vi "FaulhaberV3-Ascii_V1.vi"() -> (1 "searchnames":string[](array[string]), 2 "ID":u32[](array[numeric]), 3 "Faulhaber Objects":T3(array[cluster]))   [LabVIEW 2011] (continued)
"Default"="", "Kommentart"=""}, {"ID"=588578825, "Name"="Motor encoder_Speed filter", "type"=enum."U16", "rw"=enum."rw", "lowLimit"="0", "highLimit"="65535", "Default"="10", "Kommentart"=""}, {"ID"=588578826, "Name"="Motor encoder_Single turn position 16 bit", "type"=enum."U16", "rw"=enum."ro", "lowLimit"="", "highLimit"="", "Default"="", "Kommentart"=""}, {"ID"=588644352, "Name"="Reference encoder_Number of entries", "type"=enum."U8", "rw"=enum."ro", "lowLimit"="", "highLimit"="", "Default"="9", "Kommentart"=""}, {"ID"=588644353, "Name"="Reference encoder_Operation mode, index polarity", "type"=enum."U16", "rw"=enum."rw", "lowLimit"="0", "highLimit"="0x0107", "Default"="0x0", "Kommentart"=""}, {"ID"=588644354, "Name"="Reference encoder_IE resolution", "type"=enum."U32", "rw"=enum."rw", "lowLimit"="0", "highLimit"="4294967295", "Default"="2048", "Kommentart"=""}, {"ID"=588644355, "Name"="Reference encoder_Reference encoder position", "type"=enum."S32", "rw"=enum."ro", "lowLimit"="", "highLimit"="", "Default"="", "Kommentart"=""}, {"ID"=588644356, "Name"="Reference encoder_Gain  (numerator/divisor)", "type"=enum."S32", "rw"=enum."rw", "lowLimit"="-2147483648", "highLimit"="2147483647", "Default"="0x40004000", "Kommentart"=""}, {"ID"=588644357, "Name"="Reference encoder_RefEnc scaled position", "type"=enum."S32", "rw"=enum."rw", "lowLimit"="-2147483648", "highLimit"="2147483647", "Default"="0", "Kommentart"=""}, {"ID"=588644360, "Name"="Reference encoder_Reference encoder act speed", "type"=enum."S32", "rw"=enum."ro", "lowLimit"="", "highLimit"="", "Default"="", "Kommentart"=""}, {"ID"=588644361, "Name"="Reference encoder_Speed filter", "type"=enum."U16", "rw"=enum."rw", "lowLimit"="0", "highLimit"="65535", "Default"="10", "Kommentart"=""}, {"ID"=588709888, "Name"="PWM input_Number of entries", "type"=enum."U8", "rw"=enum."ro", "lowLimit"="", "highLimit"="", "Default"="7", "Kommentart"=""}, {"ID"=588709889, "Name"="PWM input_Digital input pin", "type"=enum."U8", "rw"=enum."unknown", "lowLimit"="", "highLimit"="", "Default"="", "Kommentart"=""}, {"ID"=588709890, "Name"="PWM input_PWM input frequency", "type"=enum."U32", "rw"=enum."ro", "lowLimit"="", "highLimit"="", "Default"="", "Kommentart"=""}, {"ID"=588709891, "Name"="PWM input_Duty cycle raw value", "type"=enum."S16", "rw"=enum."ro", "lowLimit"="", "highLimit"="", "Default"="", "Kommentart"=""}, {"ID"=588709892, "Name"="PWM input_Duty cycle  gain (numerator/divisor)", "type"=enum."U32", "rw"=enum."rw", "lowLimit"="0", "highLimit"="4294967295", "Default"="0x7FFF8000", "Kommentart"=""}, {"ID"=588709893, "Name"="PWM input_Duty cycle offset", "type"=enum."S16", "rw"=enum."rw", "lowLimit"="-32768", "highLimit"="32767", "Default"="0", "Kommentart"=""}, {"ID"=588709894, "Name"="PWM input_Duty cycle scaled value", "type"=enum."S32", "rw"=enum."ro", "lowLimit"="", "highLimit"="", "Default"="", "Kommentart"=""}, {"ID"=588709895, "Name"="PWM input_Resolution as encoder", "type"=enum."S16", "rw"=enum."rw", "lowLimit"="-32768", "highLimit"="32767", "Default"="1000", "Kommentart"=""}, {"ID"=588775424, "Name"="Hall configuration_Number of entries", "type"=enum."U8", "rw"=enum."ro", "lowLimit"="", "highLimit"="", "Default"="5", "Kommentart"=""}, {"ID"=588775425, "Name"="Hall configuration_Hall sensor type", "type"=enum."U8", "rw"=enum."ro", "lowLimit"="", "highLimit"="0x83", "Default"="", "Kommentart"=""}, {"ID"=588775426, "Name"="Hall configuration_Enable adaptation", "type"=enum."U8", "rw"=enum."rw", "lowLimit"="0", "highLimit"="255", "Default"="0", "Kommentart"=""}, {"ID"=588775427, "Name"="Hall configuration_Adaptation threshold speed", "type"=enum."U32", "rw"=enum."rw", "lowLimit"="0", "highLimit"="4294967295", "Default"="1000", "Kommentart"=""}, {"ID"=588775428, "Name"="Hall configuration_Digital hall settings of Non-Faulhaber motors", "type"=enum."U8", "rw"=enum."rw", "lowLimit"="0", "highLimit"="0x81", "Default"="0x0", "Kommentart"=""}, {"ID"=588775429, "Name"="Hall configuration_Hall filter configuration", "type"=enum."U8", "rw"=enum."rw", "lowLimit"="0", "highLimit"="0x03", "Default"="0x0", "Kommentart"=""}, {"ID"=588840960, "Name"="Reduction ratio, external position encoder_Number of entries", "type"=enum."U8", "rw"=enum."ro", "lowLimit"="", "highLimit"="", "Default"="2", "Kommentart"=""}, {"ID"=588840961, "Name"="Reduction ratio, external position encoder_Numerator", "type"=enum."U32", "rw"=enum."rw", "lowLimit"="1", "highLimit"="4294967295", "Default"="1", "Kommentart"=""}, {"ID"=588840962, "Name"="Reduction ratio, external position encoder_Divisor", "type"=enum."U32", "rw"=enum."rw", "lowLimit"="1", "highLimit"="4294967295", "Default"="1", "Kommentart"=""}, {"ID"=589234176, "Name"="231F_00_Number of entries", "type"=enum."U8", "rw"=enum."ro", "lowLimit"="", "highLimit"="", "Default"="15", "Kommentart"=""}, {"ID"=589234177, "Name"="231F_00_231F_01", "type"=enum."S16", "rw"=enum."ro", "lowLimit"="", "highLimit"="", "Default"="", "Kommentart"=""}, {"ID"=589234178, "Name"="231F_00_231F_02", "type"=enum."S16", "rw"=enum."ro", "lowLimit"="", "highLimit"="", "Default"="", "Kommentart"=""}, {"ID"=589234179, "Name"="231F_00_231F_03", "type"=enum."S16", "rw"=enum."ro", "lowLimit"="", "highLimit"="", "Default"="", "Kommentart"=""}, {"ID"=589234180, "Name"="231F_00_231F_04", "type"=enum."S16", "rw"=enum."ro", "lowLimit"="", "highLimit"="", "Default"="", "Kommentart"=""}, {"ID"=589234181, "Name"="231F_00_231F_05", "type"=enum."S16", "rw"=enum."ro", "lowLimit"="", "highLimit"="", "Default"="", "Kommentart"=""}, {"ID"=589234182, "Name"="231F_00_231F_06", "type"=enum."S16", "rw"=enum."ro", "lowLimit"="", "highLimit"="", "Default"="", "Kommentart"=""}, {"ID"=589234183, "Name"="231F_00_231F_07", "type"=enum."S16", "rw"=enum."ro", "lowLimit"="", "highLimit"="", "Default"="", "Kommentart"=""}, {"ID"=589234184, "Name"="231F_00_231F_08", "type"=enum."S16", "rw"=enum."ro", "lowLimit"="", "highLimit"="", "Default"="", "Kommentart"=""}, {"ID"=589234185, "Name"="231F_00_231F_09", "type"=enum."S16", "rw"=enum."ro", "lowLimit"="", "highLimit"="", "Default"="", "Kommentart"=""}, {"ID"=589234186, "Name"="231F_00_231F_0A", "type"=enum."S16", "rw"=enum."ro", "lowLimit"="", "highLimit"="", "Default"="", "Kommentart"=""}, {"ID"=589234187, "Name"="231F_00_231F_0B", "type"=enum."S16", "rw"=enum."ro", "lowLimit"="", "highLimit"="", "Default"="", "Kommentart"=""}, {"ID"=589234188, "Name"="231F_00_231F_0C", "type"=enum."S16", "rw"=enum."ro", "lowLimit"="", "highLimit"="", "Default"="", "Kommentart"=""}, {"ID"=589234189, "Name"="231F_00_231F_0D", "type"=enum."S16", "rw"=enum."ro", "lowLimit"="", "highLimit"="", "Default"="", "Kommentart"=""}, {"ID"=589234190, "Name"="231F_00_231F_0E", "type"=enum."S16", "rw"=enum."ro", "lowLimit"="", "highLimit"="", "Default"="", "Kommentart"=""}, {"ID"=589234191, "Name"="231F_00_231F_0F", "type"=enum."S16", "rw"=enum."ro", "lowLimit"="", "highLimit"="", "Default"="", "Kommentart"=""}, {"ID"=589299712, "Name"="Faulhaber error register", "type"=enum."U16", "rw"=enum."ro", "lowLimit"="", "highLimit"="", "Default"="", "Kommentart"=""}, {"ID"=589365248, "Name"="Error mask_Number of entries", "type"=enum."U8", "rw"=enum."ro", "lowLimit"="", "highLimit"="", "Default"="7", "Kommentart"=""}, {"ID"=589365249, "Name"="Error mask_EMCY mask", "type"=enum."U16", "rw"=enum."rw", "lowLimit"="0", "highLimit"="65535", "Default"="0xFFFF", "Kommentart"=""}, {"ID"=589365250, "Name"="Error mask_Fault mask", "type"=enum."U16", "rw"=enum."rw", "lowLimit"="0", "highLimit"="0xBFD3", "Default"="0x0000", "Kommentart"=""}, {"ID"=589365251, "Name"="Error mask_Error out mask", "type"=enum."U16", "rw"=enum."rw", "lowLimit"="0", "highLimit"="65535", "Default"="0x0000", "Kommentart"=""}, {"ID"=589365252, "Name"="Error mask_Disable voltage mask manufacturer", "type"=enum."U16", "rw"=enum."ro", "lowLimit"="", "highLimit"="", "Default"="0x402C", "Kommentart"=""}, {"ID"=589365253, "Name"="Error mask_Disable voltage mask user", "type"=enum."U16", "rw"=enum."rw", "lowLimit"="0", "highLimit"="0xBFD3", "Default"="0x0000", "Kommentart"=""}, {"ID"=589365254, "Name"="Error mask_Quick stop mask", "type"=enum."U16", "rw"=enum."rw", "lowLimit"="0", "highLimit"="0xBFD3", "Default"="0x0000", "Kommentart"=""}, {"ID"=589365255, "Name"="Error mask_Error bit mask", "type"=enum."U16", "rw"=enum."rw", "lowLimit"="0", "highLimit"="65535", "Default"="0x0000", "Kommentart"=""}, {"ID"=589430784, "Name"="Error codes_Number of entries", "type"=enum."U8", "rw"=enum."ro", "lowLimit"="", "highLimit"="", "Default"="1", "Kommentart"=""}, {"ID"=589430785, "Name"="Error codes_ScriptingError", "type"=enum."U16", "rw"=enum."ro", "lowLimit"="", "highLimit"="", "Default"="0", "Kommentart"=""}, {"ID"=589561856, "Name"="Device status_Number of entries", "type"=enum."U8", "rw"=enum."ro", "lowLimit"="", "highLimit"="", "Default"="9", "Kommentart"=""}, {"ID"=589561857, "Name"="Device status_Device status word", "type"=enum."U32", "rw"=enum."ro", "lowLimit"="0x0", "highLimit"="", "Default"="", "Kommentart"=""}, {"ID"=589561858, "Name"="Device status_Limit check delay time", "type"=enum."U16", "rw"=enum."rw", "lowLimit"="0", "highLimit"="65535", "Default"="10", "Kommentart"=""}, {"ID"=589561859, "Name"="Device status_Reserved 3", "type"=enum."U8", "rw"=enum."ro", "lowLimit"="", "highLimit"="", "Default"="", "Kommentart"=""}, {"ID"=589561860, "Name"="Device status_Reserved 4", "type"=enum."S16", "rw"=enum."ro", "lowLimit"="", "highLimit"="", "Default"="", "Kommentart"=""}, {"ID"=589561861, "Name"="Device status_Reserved 5", "type"=enum."S16", "rw"=enum."ro", "lowLimit"="", "highLimit"="", "Default"="", "Kommentart"=""}, {"ID"=589561862, "Name"="Device status_Reserved 6", "type"=enum."S32", "rw"=enum."ro", "lowLimit"="", "highLimit"="", "Default"="", "Kommentart"=""}, {"ID"=589561863, "Name"="Device status_Reserved 7", "type"=enum."S32", "rw"=enum."ro", "lowLimit"="", "highLimit"="", "Default"="", "Kommentart"=""}, {"ID"=589561864, "Name"="Device status_Reserved 8", "type"=enum."U8", "rw"=enum."wo", "lowLimit"="0", "highLimit"="255", "Default"="", "Kommentart"=""}, {"ID"=589561865, "Name"="Device status_Reserved 9", "type"=enum."U8", "rw"=enum."wo", "lowLimit"="0", "highLimit"="255", "Default"="", "Kommentart"=""}, {"ID"=589627392, "Name"="Voltage monitor_Number of entries", "type"=enum."U8", "rw"=enum."ro", "lowLimit"="", "highLimit"="", "Default"="7", "Kommentart"=""}, {"ID"=589627393, "Name"="Voltage monitor_Device supply lower threshold", "type"=enum."U16", "rw"=enum."ro", "lowLimit"="", "highLimit"="", "Default"="", "Kommentart"=""}, {"ID"=589627394, "Name"="Voltage monitor_Motor supply lower threshold", "type"=enum."U16", "rw"=enum."rw", "lowLimit"="0", "highLimit"="65535", "Default"="", "Kommentart"=""}, {"ID"=589627395, "Name"="Voltage monitor_Motor supply max threshold", "type"=enum."U16", "rw"=enum."ro", "lowLimit"="", "highLimit"="", "Default"="", "Kommentart"=""}, {"ID"=589627396, "Name"="Voltage monitor_Motor supply upper threshold", "type"=enum."U16", "rw"=enum."rw", "lowLimit"="0", "highLimit"="65535", "Default"="", "Kommentart"=""}, {"ID"=589627397, "Name"="Voltage monitor_Voltage error delay time", "type"=enum."U16", "rw"=enum."rw", "lowLimit"="0", "highLimit"="65535", "Default"="200", "Kommentart"=""}, {"ID"=589627398, "Name"="Voltage monitor_Device supply voltage", "type"=enum."U16", "rw"=enum."ro", "lowLimit"="", "highLimit"="", "Default"="", "Kommentart"=""}, {"ID"=589627399, "Name"="Voltage monitor_Motor supply voltage", "type"=enum."U16", "rw"=enum."ro", "lowLimit"="", "highLimit"="", "Default"="", "Kommentart"=""}, {"ID"=589692928, "Name"="Device temperature_Number of entries", "type"=enum."U8", "rw"=enum."ro", "lowLimit"="", "highLimit"="", "Default"="11", "Kommentart"=""}, {"ID"=589692929, "Name"="Device temperature_CPU temperature", "type"=enum."S16", "rw"=enum."ro", "lowLimit"="", "highLimit"="", "Default"="", "Kommentart"=""}, {"ID"=589692930, "Name"="Device temperature_Power stage temperature", "type"=enum."S16", "rw"=enum."ro", "lowLimit"="", "highLimit"="", "Default"="", "Kommentart"=""}, {"ID"=589692931, "Name"="Device temperature_Winding temperature", "type"=enum."S16", "rw"=enum."ro", "lowLimit"="", "highLimit"="", "Default"="", "Kommentart"=""}, {"ID"=589692932, "Name"="Device temperature_CPU temperature shutdown threshold", "type"=enum."S16", "rw"=enum."ro", "lowLimit"="", "highLimit"="", "Default"="", "Kommentart"=""}, {"ID"=589692933, "Name"="Device temperature_CPU temperature warning threshold", "type"=enum."S16", "rw"=enum."ro", "lowLimit"="", "highLimit"="", "Default"="", "Kommentart"=""}, {"ID"=589692934, "Name"="Device temperature_Power stage temperature shutdown threshold", "type"=enum."S16", "rw"=enum."ro", "lowLimit"="", "highLimit"="", "Default"="", "Kommentart"=""}, {"ID"=589692935, "Name"="Device temperature_Power stage temperature warning threshold", "type"=enum."S16", "rw"=enum."ro", "lowLimit"="", "highLimit"="", "Default"="", "Kommentart"=""}, {"ID"=589692936, "Name"="Device temperature_Winding temperature shutdown threshold", "type"=enum."S16", "rw"=enum."rw", "lowLimit"="-32768", "highLimit"="32767", "Default"="", "Kommentart"=""}, {"ID"=589692937, "Name"="Device temperature_Winding temperature warning threshold", "type"=enum."S16", "rw"=enum."rw", "lowLimit"="-32768", "highLimit"="32767", "Default"="", "Kommentart"=""}, {"ID"=589692938, "Name"="Device temperature_Motor NTC temperature", "type"=enum."S16", "rw"=enum."ro", "lowLimit"="", "highLimit"="", "Default"="", "Kommentart"=""}, {"ID"=589692939, "Name"="Device temperature_Motor NTC enable", "type"=enum."S16", "rw"=enum."ro", "lowLimit"="0", "highLimit"="1", "Default"="1", "Kommentart"=""}, {"ID"=589758464, "Name"="Device data_Number of entries", "type"=enum."U8", "rw"=enum."ro", "lowLimit"="", "highLimit"="", "Default"="3", "Kommentart"=""}, {"ID"=589758465, "Name"="Device data_Device nominal current", "type"=enum."U16", "rw"=enum."ro", "lowLimit"="1000", "highLimit"="5000", "Default"="", "Kommentart"=""}, {"ID"=589758466, "Name"="Device data_Device peak current", "type"=enum."U16", "rw"=enum."ro", "lowLimit"="", "highLimit"="", "Default"="", "Kommentart"=""}, {"ID"=589758467, "Name"="Device data_Device nominal voltage", "type"=enum."U16", "rw"=enum."ro", "lowLimit"="", "highLimit"="", "Default"="", "Kommentart"=""}, {"ID"=589824000, "Name"="Device data for thermal model_Number of entries", "type"=enum."U8", "rw"=enum."ro", "lowLimit"="", "highLimit"="", "Default"="9", "Kommentart"=""}, {"ID"=589824001, "Name"="Device data for thermal model_Controller type", "type"=enum."U8", "rw"=enum."unknown", "lowLimit"="", "highLimit"="", "Default"="", "Kommentart"=""}, {"ID"=589824002, "Name"="Device data for thermal model_Power stage Rdson", "type"=enum."U8", "rw"=enum."ro", "lowLimit"="", "highLimit"="", "Default"="", "Kommentart"=""}, {"ID"=589824003, "Name"="Device data for thermal model_Power stage LossFactor", "type"=enum."U16", "rw"=enum."ro", "lowLimit"="", "highLimit"="", "Default"="", "Kommentart"=""}, {"ID"=589824004, "Name"="Device data for thermal model_Power stage Rth1", "type"=enum."U16", "rw"=enum."ro", "lowLimit"="", "highLimit"="", "Default"="", "Kommentart"=""}, {"ID"=589824005, "Name"="Device data for thermal model_Power stage Time Constant 1", "type"=enum."U16", "rw"=enum."ro", "lowLimit"="", "highLimit"="", "Default"="", "Kommentart"=""}, {"ID"=589824006, "Name"="Device data for thermal model_Power stage Rth2", "type"=enum."U16", "rw"=enum."ro", "lowLimit"="", "highLimit"="", "Default"="", "Kommentart"=""}, {"ID"=589824007, "Name"="Device data for thermal model_Power stage Time Constant 2", "type"=enum."U16", "rw"=enum."ro", "lowLimit"="", "highLimit"="", "Default"="", "Kommentart"=""}, {"ID"=589824008, "Name"="Device data for thermal model_Power stage Rth3", "type"=enum."U16", "rw"=enum."ro", "lowLimit"="", "highLimit"="", "Default"="", "Kommentart"=""}, {"ID"=589824009, "Name"="Device data for thermal model_Power stage Rth4", "type"=enum."U16", "rw"=enum."ro", "lowLimit"="", "highLimit"="", "Default"="", "Kommentart"=""}, {"ID"=589889536, "Name"="Motor and application data for motor control_Number of entries", "type"=enum."U8", "rw"=enum."ro", "lowLimit"="", "highLimit"="", "Default"="18", "Kommentart"=""}, {"ID"=589889537, "Name"="Motor and application data for motor control_Rated current", "type"=enum."U16", "rw"=enum."rw", "lowLimit"="0", "highLimit"="65535", "Default"="", "Kommentart"=""}, {"ID"=589889538, "Name"="Motor and application data for motor control_Continous current", "type"=enum."U16", "rw"=enum."rw", "lowLimit"="0", "highLimit"="65535", "Default"="", "Kommentart"=""}, {"ID"=589889539, "Name"="Motor and application data for motor control_Peak current", "type"=enum."U16", "rw"=enum."rw", "lowLimit"="0", "highLimit"="65535", "Default"="", "Kommentart"=""}, {"ID"=589889540, "Name"="Motor and application data for motor control_Torque constant / Force constant", "type"=enum."U32", "rw"=enum."rw", "lowLimit"="0", "highLimit"="3500000", "Default"="", "Kommentart"=""}, {"ID"=589889541, "Name"="Motor and application data for motor control_Terminal inductance", "type"=enum."U32", "rw"=enum."rw", "lowLimit"="0", "highLimit"="200000", "Default"="", "Kommentart"=""}, {"ID"=589889542, "Name"="Motor and application data for motor control_Inductance Ld", "type"=enum."U32", "rw"=enum."rw", "lowLimit"="0", "highLimit"="200000", "Default"="", "Kommentart"=""}, {"ID"=589889543, "Name"="Motor and application data for motor control_Number of pole pairs", "type"=enum."U8", "rw"=enum."ro", "lowLimit"="", "highLimit"="", "Default"="", "Kommentart"=""}, {"ID"=589889544, "Name"="Motor and application data for motor control_Phase angle offset", "type"=enum."S16", "rw"=enum."rw", "lowLimit"="-32768", "highLimit"="32767", "Default"="", "Kommentart"=""}, {"ID"=589889545, "Name"="Motor and application data for motor control_Rotor inertia / Rod weight", "type"=enum."U32", "rw"=enum."rw", "lowLimit"="0", "highLimit"="4294967295", "Default"="", "Kommentart"=""}, {"ID"=589889546, "Name"="Motor and application data for motor control_Load inertia / Load mass", "type"=enum."U32", "rw"=enum."rw", "lowLimit"="0", "highLimit"="4294967295", "Default"="", "Kommentart"=""}, {"ID"=589889547, "Name"="Motor and application data for motor control_Motor type", "type"=enum."U8", "rw"=enum."unknown", "lowLimit"="", "highLimit"="", "Default"="", "Kommentart"=""}, {"ID"=589889548, "Name"="Motor and application data for motor control_Magnetic pitch of linear motor", "type"=enum."U8", "rw"=enum."rw", "lowLimit"="0", "highLimit"="60", "Default"="", "Kommentart"=""}, {"ID"=589889549, "Name"="Motor and application data for motor control_Filter phase inductance", "type"=enum."U8", "rw"=enum."rw", "lowLimit"="0", "highLimit"="255", "Default"="", "Kommentart"=""}, {"ID"=589889550, "Name"="Motor and application data for motor control_Factor speed constant", "type"=enum."U16", "rw"=enum."rw", "lowLimit"="750", "highLimit"="1250", "Default"="", "Kommentart"=""}, {"ID"=589889551, "Name"="Motor and application data for motor control_Steps per turn", "type"=enum."U16", "rw"=enum."rw", "lowLimit"="0", "highLimit"="65535", "Default"="24", "Kommentart"=""}, {"ID"=589889552, "Name"="Motor and application data for motor control_Stepper interpolation factor", "type"=enum."U16", "rw"=enum."rw", "lowLimit"="0", "highLimit"="65535", "Default"="512", "Kommentart"=""}, {"ID"=589889553, "Name"="Motor and application data for motor control_Stepper current reduction at n=0", "type"=enum."U8", "rw"=enum."rw", "lowLimit"="0", "highLimit"="100", "Default"="60", "Kommentart"=""}, {"ID"=589889554, "Name"="Motor and application data for motor control_Current holding time at n=0", "type"=enum."U16", "rw"=enum."rw", "lowLimit"="0", "highLimit"="65535", "Default"="200", "Kommentart"=""}, {"ID"=589955072, "Name"="Motor and application data for thermal motor model_Number of entries", "type"=enum."U8", "rw"=enum."ro", "lowLimit"="", "highLimit"="", "Default"="10", "Kommentart"=""}, {"ID"=589955073, "Name"="Motor and application data for thermal motor model_Terminal resistance", "type"=enum."U32", "rw"=enum."rw", "lowLimit"="0", "highLimit"="4294967295", "Default"="", "Kommentart"=""}, {"ID"=589955074, "Name"="Motor and application data for thermal motor model_Friction", "type"=enum."U32", "rw"=enum."rw", "lowLimit"="0", "highLimit"="4294967295", "Default"="", "Kommentart"=""}, {"ID"=589955075, "Name"="Motor and application data for thermal motor model_Friction,dynamic", "type"=enum."U32", "rw"=enum."rw", "lowLimit"="0", "highLimit"="4294967295", "Default"="", "Kommentart"=""}, {"ID"=589955076, "Name"="Motor and application data for thermal motor model_Thermal resistance 1", "type"=enum."U16", "rw"=enum."rw", "lowLimit"="0", "highLimit"="65535", "Default"="", "Kommentart"=""}, {"ID"=589955077, "Name"="Motor and application data for thermal motor model_Thermal resistance 2", "type"=enum."U32", "rw"=enum."rw", "lowLimit"="0", "highLimit"="4294967295", "Default"="", "Kommentart"=""}, {"ID"=589955078, "Name"="Motor and application data for thermal motor model_Thermal time constant 1", "type"=enum."U16", "rw"=enum."rw", "lowLimit"="0", "highLimit"="65535", "Default"="", "Kommentart"=""}, {"ID"=589955079, "Name"="Motor and application data for thermal motor model_Thermal time constant 2", "type"=enum."U16", "rw"=enum."rw", "lowLimit"="0", "highLimit"="65535", "Default"="", "Kommentart"=""}, {"ID"=589955080, "Name"="Motor and application data for thermal motor model_Ambient temperature", "type"=enum."U8", "rw"=enum."rw", "lowLimit"="0", "highLimit"="255", "Default"="22", "Kommentart"=""}, {"ID"=589955081, "Name"="Motor and application data for thermal motor model_Reduction of thermal resistance 2", "type"=enum."U8", "rw"=enum."rw", "lowLimit"="0", "highLimit"="99", "Default"="25", "Kommentart"=""}, {"ID"=589955082, "Name"="Motor and application data for thermal motor model_Selection of thermal model", "type"=enum."U8", "rw"=enum."rw", "lowLimit"="0", "highLimit"="2", "Default"="0", "Kommentart"=""}, {"ID"=590020608, "Name"="Motor alignment parameters_Number of entries", "type"=enum."U8", "rw"=enum."ro", "lowLimit"="", "highLimit"="", "Default"="5", "Kommentart"=""}, {"ID"=590020609, "Name"="Motor alignment parameters_Setup time", "type"=enum."U16", "rw"=enum."rw", "lowLimit"="0", "highLimit"="65535", "Default"="5", "Kommentart"=""}, {"ID"=590020610, "Name"="Motor alignment parameters_Delta time step 1", "type"=enum."U16", "rw"=enum."rw", "lowLimit"="0", "highLimit"="65535", "Default"="250", "Kommentart"=""}, {"ID"=590020611, "Name"="Motor alignment parameters_Delta time step 2", "type"=enum."U16", "rw"=enum."rw", "lowLimit"="0", "highLimit"="65535", "Default"="250", "Kommentart"=""}, {"ID"=590020612, "Name"="Motor alignment parameters_Delta time step 3", "type"=enum."U16", "rw"=enum."rw", "lowLimit"="0", "highLimit"="65535", "Default"="250", "Kommentart"=""}, {"ID"=590020613, "Name"="Motor alignment parameters_Delta postion tolerance", "type"=enum."U16", "rw"=enum."rw", "lowLimit"="0", "highLimit"="65535", "Default"="4096", "Kommentart"=""}, {"ID"=590086144, "Name"="Motor alignment results_Number of entries", "type"=enum."U8", "rw"=enum."ro", "lowLimit"="", "highLimit"="", "Default"="3", "Kommentart"=""}, {"ID"=590086145, "Name"="Motor alignment results_Position A1", "type"=enum."U16", "rw"=enum."ro", "lowLimit"="", "highLimit"="", "Default"="", "Kommentart"=""}, {"ID"=590086146, "Name"="Motor alignment results_Position B", "type"=enum."U16", "rw"=enum."ro", "lowLimit"="", "highLimit"="", "Default"="", "Kommentart"=""}, {"ID"=590086147, "Name"="Motor alignment results_Position A2", "type"=enum."U16", "rw"=enum."ro", "lowLimit"="", "highLimit"="", "Default"="", "Kommentart"=""}, {"ID"=590348288, "Name"="Switch position for actual values _Number of entries", "type"=enum."U8", "rw"=enum."ro", "lowLimit"="", "highLimit"="", "Default"="3", "Kommentart"=""}, {"ID"=590348289, "Name"="Switch position for actual values _Actual commutation angle source", "type"=enum."U8", "rw"=enum."unknown", "lowLimit"="", "highLimit"="", "Default"="", "Kommentart"=""}, {"ID"=590348290, "Name"="Switch position for actual values _Actual velocity source", "type"=enum."U8", "rw"=enum."unknown", "lowLimit"="", "highLimit"="", "Default"="", "Kommentart"=""}, {"ID"=590348291, "Name"="Switch position for actual values _Actual position source", "type"=enum."U8", "rw"=enum."unknown", "lowLimit"="", "highLimit"="", "Default"="", "Kommentart"=""}, {"ID"=590413824, "Name"="Discrete sources_Number of entries", "type"=enum."U8", "rw"=enum."ro", "lowLimit"="", "highLimit"="", "Default"="4", "Kommentart"=""}, {"ID"=590413825, "Name"="Discrete sources_Target voltage source", "type"=enum."U8", "rw"=enum."unknown", "lowLimit"="", "highLimit"="", "Default"="", "Kommentart"=""}, {"ID"=590413826, "Name"="Discrete sources_Target current source", "type"=enum."U8", "rw"=enum."unknown", "lowLimit"="", "highLimit"="", "Default"="", "Kommentart"=""}, {"ID"=590413827, "Name"="Discrete sources_Target velocity source", "type"=enum."U8", "rw"=enum."unknown", "lowLimit"="", "highLimit"="", "Default"="", "Kommentart"=""}, {"ID"=590413828, "Name"="Discrete sources_Target position source", "type"=enum."U8", "rw"=enum."unknown", "lowLimit"="", "highLimit"="", "Default"="", "Kommentart"=""}, {"ID"=590479360, "Name"="Cyclic mode interpolation rate ", "type"=enum."U16", "rw"=enum."rw", "lowLimit"="1", "highLimit"="65535", "Default"="1", "Kommentart"=""}, {"ID"=591003648, "Name"="Manufacturer specified bits_Number of entries", "type"=enum."U8", "rw"=enum."ro", "lowLimit"="", "highLimit"="", "Default"="2", "Kommentart"=""}, {"ID"=591003649, "Name"="Manufacturer specified bits_Bit mask for bit 14", "type"=enum."U32", "rw"=enum."rw", "lowLimit"="0", "highLimit"="4294967295", "Default"="0x0", "Kommentart"=""}, {"ID"=591003650, "Name"="Manufacturer specified bits_Bit mask for bit 15", "type"=enum."U32", "rw"=enum."rw", "lowLimit"="0", "highLimit"="4294967295", "Default"="0x0", "Kommentart"=""}, {"ID"=591265792, "Name"="Selection of controller scaling", "type"=enum."U8", "rw"=enum."rw", "lowLimit"="0", "highLimit"="255", "Default"="0x00", "Kommentart"=""}, {"ID"=591331328, "Name"="Operation mode options", "type"=enum."U16", "rw"=enum."rw", "lowLimit"="0x0", "highLimit"="0x80FF", "Default"="", "Kommentart"=""}, {"ID"=591396864, "Name"="General parameters_Number of entries", "type"=enum."U8", "rw"=enum."ro", "lowLimit"="", "highLimit"="", "Default"="9", "Kommentart"=""}, {"ID"=591396865, "Name"="General parameters_Commutation type", "type"=enum."U8", "rw"=enum."unknown", "lowLimit"="", "highLimit"="", "Default"="", "Kommentart"=""}, {"ID"=591396866, "Name"="General parameters_Motor output voltage DC", "type"=enum."S16", "rw"=enum."rw", "lowLimit"="-32768", "highLimit"="32767", "Default"="0", "Kommentart"=""}, {"ID"=591396867, "Name"="General parameters_Motor output voltage BL block", "type"=enum."S16", "rw"=enum."rw", "lowLimit"="-32768", "highLimit"="32767", "Default"="0", "Kommentart"=""}, {"ID"=591396868, "Name"="General parameters_Motor output voltage Xd", "type"=enum."S16", "rw"=enum."rw", "lowLimit"="-32768", "highLimit"="32767", "Default"="0", "Kommentart"=""}, {"ID"=591396869, "Name"="General parameters_Motor output voltage Xq", "type"=enum."S16", "rw"=enum."rw", "lowLimit"="-32768", "highLimit"="32767", "Default"="0", "Kommentart"=""}, {"ID"=591396870, "Name"="General parameters_Sinus output voltage Ua", "type"=enum."U16", "rw"=enum."ro", "lowLimit"="", "highLimit"="", "Default"="", "Kommentart"=""}, {"ID"=591396871, "Name"="General parameters_Sinus output voltage Ub", "type"=enum."U16", "rw"=enum."ro", "lowLimit"="", "highLimit"="", "Default"="", "Kommentart"=""}, {"ID"=591396872, "Name"="General parameters_Sinus output voltage Uc", "type"=enum."U16", "rw"=enum."ro", "lowLimit"="", "highLimit"="", "Default"="", "Kommentart"=""}, {"ID"=591396873, "Name"="General parameters_Sinus output voltage Ud", "type"=enum."U16", "rw"=enum."ro", "lowLimit"="", "highLimit"="", "Default"="", "Kommentart"=""}, {"ID"=591462400, "Name"="Target voltage", "type"=enum."S16", "rw"=enum."rw", "lowLimit"="-32768", "highLimit"="32767", "Default"="0", "Kommentart"=""}, {"ID"=591527936, "Name"="Torque control parameters_Number of entries", "type"=enum."U8", "rw"=enum."ro", "lowLimit"="", "highLimit"="", "Default"="2", "Kommentart"=""}, {"ID"=591527937, "Name"="Torque control parameters_Gain Kpi", "type"=enum."U32", "rw"=enum."rw", "lowLimit"="0", "highLimit"="4294967295", "Default"="", "Kommentart"=""}, {"ID"=591527938, "Name"="Torque control parameters_Integral time Tni", "type"=enum."U16", "rw"=enum."rw", "lowLimit"="150", "highLimit"="2600", "Default"="", "Kommentart"=""}, {"ID"=591593472, "Name"="Flux control parameters_Number of entries", "type"=enum."U8", "rw"=enum."ro", "lowLimit"="", "highLimit"="", "Default"="2", "Kommentart"=""}, {"ID"=591593473, "Name"="Flux control parameters_Gain Kpi", "type"=enum."U32", "rw"=enum."rw", "lowLimit"="0", "highLimit"="4294967295", "Default"="", "Kommentart"=""}, {"ID"=591593474, "Name"="Flux control parameters_Integral time Tni", "type"=enum."U16", "rw"=enum."rw", "lowLimit"="150", "highLimit"="2600", "Default"="", "Kommentart"=""}, {"ID"=591659008, "Name"="Velocity control parameters_Number of entries", "type"=enum."U8", "rw"=enum."ro", "lowLimit"="", "highLimit"="", "Default"="6", "Kommentart"=""}, {"ID"=591659009, "Name"="Velocity control parameters_Gain KP", "type"=enum."U32", "rw"=enum."rw", "lowLimit"="0", "highLimit"="4294967295", "Default"="", "Kommentart"=""}, {"ID"=591659010, "Name"="Velocity control parameters_Integral time TN", "type"=enum."U16", "rw"=enum."rw", "lowLimit"="20", "highLimit"="1000", "Default"="", "Kommentart"=""}, {"ID"=591659011, "Name"="Velocity control parameters_Velocity deviation threshold", "type"=enum."U16", "rw"=enum."rw", "lowLimit"="0", "highLimit"="65535", "Default"="65535", "Kommentart"=""}, {"ID"=591659012, "Name"="Velocity control parameters_Velocity deviation time", "type"=enum."U16", "rw"=enum."rw", "lowLimit"="1", "highLimit"="65535", "Default"="100", "Kommentart"=""}, {"ID"=591659013, "Name"="Velocity control parameters_Velocity warning threshold", "type"=enum."U32", "rw"=enum."rw", "lowLimit"="1", "highLimit"="0x007FFFFF", "Default"="30000", "Kommentart"=""}, {"ID"=591659014, "Name"="Velocity control parameters_Integral part option", "type"=enum."U8", "rw"=enum."unknown", "lowLimit"="", "highLimit"="", "Default"="", "Kommentart"=""}, {"ID"=591724544, "Name"="Velocity filter parameters_Number of entries", "type"=enum."U8", "rw"=enum."ro", "lowLimit"="", "highLimit"="", "Default"="2", "Kommentart"=""}, {"ID"=591724545, "Name"="Velocity filter parameters_Actual velocity filter TF", "type"=enum."U16", "rw"=enum."rw", "lowLimit"="0", "highLimit"="65535", "Default"="", "Kommentart"=""}, {"ID"=591724546, "Name"="Velocity filter parameters_Display velocity filter", "type"=enum."U16", "rw"=enum."rw", "lowLimit"="0", "highLimit"="65535", "Default"="", "Kommentart"=""}, {"ID"=591790080, "Name"="Setpoint velocity filter parameters_Number of entries", "type"=enum."U8", "rw"=enum."ro", "lowLimit"="", "highLimit"="", "Default"="2", "Kommentart"=""}, {"ID"=591790081, "Name"="Setpoint velocity filter parameters_Setpoint velocity filter TF", "type"=enum."U16", "rw"=enum."rw", "lowLimit"="0", "highLimit"="65535", "Default"="", "Kommentart"=""}, {"ID"=591790082, "Name"="Setpoint velocity filter parameters_Setpoint filter enable", "type"=enum."U8", "rw"=enum."unknown", "lowLimit"="", "highLimit"="", "Default"="", "Kommentart"=""}, {"ID"=591855616, "Name"="Gain scheduling_Number of entries", "type"=enum."U8", "rw"=enum."ro", "lowLimit"="", "highLimit"="", "Default"="2", "Kommentart"=""}, {"ID"=591855617, "Name"="Gain scheduling_Gain factor Kpn", "type"=enum."U8", "rw"=enum."rw", "lowLimit"="0", "highLimit"="255", "Default"="128", "Kommentart"=""}, {"ID"=591855618, "Name"="Gain scheduling_Gain factor Kv", "type"=enum."U8", "rw"=enum."rw", "lowLimit"="0", "highLimit"="255", "Default"="128", "Kommentart"=""}, {"ID"=591921152, "Name"="Position control parameters_Number of entries", "type"=enum."U8", "rw"=enum."ro", "lowLimit"="", "highLimit"="", "Default"="1", "Kommentart"=""}, {"ID"=591921153, "Name"="Position control parameters_Gain Kv", "type"=enum."U8", "rw"=enum."rw", "lowLimit"="0", "highLimit"="255", "Default"="", "Kommentart"=""}, {"ID"=591986688, "Name"="Current feedforward parameters_Number of entries", "type"=enum."U8", "rw"=enum."ro", "lowLimit"="", "highLimit"="", "Default"="2", "Kommentart"=""}, {"ID"=591986689, "Name"="Current feedforward parameters_Current feedforward factor", "type"=enum."U8", "rw"=enum."rw", "lowLimit"="0", "highLimit"="128", "Default"="0", "Kommentart"=""}, {"ID"=591986690, "Name"="Current feedforward parameters_Current feedforward delay", "type"=enum."U16", "rw"=enum."rw", "lowLimit"="0", "highLimit"="65535", "Default"="0", "Kommentart"=""}, {"ID"=592052224, "Name"="Velocity feedforward parameters_Number of entries", "type"=enum."U8", "rw"=enum."ro", "lowLimit"="", "highLimit"="", "Default"="2", "Kommentart"=""}, {"ID"=592052225, "Name"="Velocity feedforward parameters_Velocity feedforward factor", "type"=enum."U8", "rw"=enum."rw", "lowLimit"="0", "highLimit"="128", "Default"="0", "Kommentart"=""}, {"ID"=592052226, "Name"="Velocity feedforward parameters_Velocity feedforward delay", "type"=enum."U16", "rw"=enum."rw", "lowLimit"="0", "highLimit"="65535", "Default"="0", "Kommentart"=""}, {"ID"=592117760, "Name"="Current filter parameters_Number of entries", "type"=enum."U8", "rw"=enum."ro", "lowLimit"="", "highLimit"="", "Default"="2", "Kommentart"=""}, {"ID"=592117761, "Name"="Current filter parameters_Display current filter TF", "type"=enum."U16", "rw"=enum."rw", "lowLimit"="0", "highLimit"="65535", "Default"="", "Kommentart"=""}, {"ID"=592117762, "Name"="Current filter parameters_Display torque filter TF", "type"=enum."U16", "rw"=enum."rw", "lowLimit"="0", "highLimit"="65535", "Default"="", "Kommentart"=""}, {"ID"=592183296, "Name"="Current compensation parameters_Number of entries", "type"=enum."U8", "rw"=enum."ro", "lowLimit"="", "highLimit"="", "Default"="3", "Kommentart"=""}, {"ID"=592183297, "Name"="Current compensation parameters_Gravity compensation", "type"=enum."S16", "rw"=enum."rw", "lowLimit"="-32768", "highLimit"="32767", "Default"="0", "Kommentart"=""}, {"ID"=592183298, "Name"="Current compensation parameters_Positive friction compensation", "type"=enum."U16", "rw"=enum."rw", "lowLimit"="0", "highLimit"="6000", "Default"="0", "Kommentart"=""}, {"ID"=592183299, "Name"="Current compensation parameters_Negative friction compensation", "type"=enum."U16", "rw"=enum."rw", "lowLimit"="0", "highLimit"="6000", "Default"="0", "Kommentart"=""}, {"ID"=592445440, "Name"="Positive torque limit homing", "type"=enum."U16", "rw"=enum."rw", "lowLimit"="0", "highLimit"="6000", "Default"="1000", "Kommentart"=""}, {"ID"=592510976, "Name"="Negative torque limit homing", "type"=enum."U16", "rw"=enum."rw", "lowLimit"="0", "highLimit"="6000", "Default"="1000", "Kommentart"=""}, {"ID"=593494016, "Name"="Actual values_Number of entries", "type"=enum."U8", "rw"=enum."ro", "lowLimit"="", "highLimit"="", "Default"="10", "Kommentart"=""}, {"ID"=593494017, "Name"="Actual values_Motor current Id actual value", "type"=enum."S16", "rw"=enum."ro", "lowLimit"="", "highLimit"="", "Default"="", "Kommentart"=""}, {"ID"=593494018, "Name"="Actual values_Motor current Iq actual value", "type"=enum."S16", "rw"=enum."ro", "lowLimit"="", "highLimit"="", "Default"="", "Kommentart"=""}, {"ID"=593494019, "Name"="Actual values_Motor currrent IBlock actual value", "type"=enum."S16", "rw"=enum."ro", "lowLimit"="", "highLimit"="", "Default"="", "Kommentart"=""}, {"ID"=593494020, "Name"="Actual values_Motor current IDC actual value", "type"=enum."S16", "rw"=enum."ro", "lowLimit"="", "highLimit"="", "Default"="", "Kommentart"=""}, {"ID"=593494021, "Name"="Actual values_Velocity actual internal value", "type"=enum."S16", "rw"=enum."ro", "lowLimit"="", "highLimit"="", "Default"="", "Kommentart"=""}, {"ID"=593494022, "Name"="Actual values_Position actual internal value", "type"=enum."S32", "rw"=enum."ro", "lowLimit"="", "highLimit"="", "Default"="", "Kommentart"=""}, {"ID"=593494023, "Name"="Actual values_Actual commutation segment", "type"=enum."U8", "rw"=enum."ro", "lowLimit"="", "highLimit"="", "Default"="", "Kommentart"=""}, {"ID"=593494024, "Name"="Actual values_Actual commutation angle", "type"=enum."S16", "rw"=enum."ro", "lowLimit"="", "highLimit"="", "Default"="", "Kommentart"=""}, {"ID"=593494025, "Name"="Actual values_Reserved 9", "type"=enum."S32", "rw"=enum."ro", "lowLimit"="", "highLimit"="", "Default"="", "Kommentart"=""}, {"ID"=593494026, "Name"="Actual values_Reserved 10", "type"=enum."S32", "rw"=enum."wo", "lowLimit"="-2147483648", "highLimit"="2147483647", "Default"="", "Kommentart"=""}, {"ID"=594542592, "Name"="Trace configuration_Number of entries", "type"=enum."U8", "rw"=enum."ro", "lowLimit"="", "highLimit"="", "Default"="15", "Kommentart"=""}, {"ID"=594542593, "Name"="Trace configuration_Trigger value", "type"=enum."U32", "rw"=enum."rw", "lowLimit"="0", "highLimit"="4294967295", "Default"="0x00", "Kommentart"=""}, {"ID"=594542594, "Name"="Trace configuration_Trigger threshold", "type"=enum."S32", "rw"=enum."rw", "lowLimit"="-2147483648", "highLimit"="2147483647", "Default"="0", "Kommentart"=""}, {"ID"=594542595, "Name"="Trace configuration_Trigger offset", "type"=enum."S16", "rw"=enum."rw", "lowLimit"="-32768", "highLimit"="32767", "Default"="0", "Kommentart"=""}, {"ID"=594542596, "Name"="Trace configuration_Trigger mode", "type"=enum."U16", "rw"=enum."rw", "lowLimit"="0", "highLimit"="65535", "Default"="0", "Kommentart"=""}, {"ID"=594542597, "Name"="Trace configuration_Buffer length", "type"=enum."U16", "rw"=enum."rw", "lowLimit"="1", "highLimit"="2048", "Default"="2048", "Kommentart"=""}, {"ID"=594542598, "Name"="Trace configuration_Sample time", "type"=enum."U8", "rw"=enum."rw", "lowLimit"="1", "highLimit"="255", "Default"="1", "Kommentart"=""}, {"ID"=594542599, "Name"="Trace configuration_Trace source of channel 1", "type"=enum."U32", "rw"=enum."rw", "lowLimit"="0", "highLimit"="4294967295", "Default"="0x00", "Kommentart"=""}, {"ID"=594542600, "Name"="Trace configuration_Trace source of channel 2", "type"=enum."U32", "rw"=enum."rw", "lowLimit"="0", "highLimit"="4294967295", "Default"="0x00", "Kommentart"=""}, {"ID"=594542601, "Name"="Trace configuration_Trace source of channel 3", "type"=enum."U32", "rw"=enum."rw", "lowLimit"="0", "highLimit"="4294967295", "Default"="0x00", "Kommentart"=""}, {"ID"=594542602, "Name"="Trace configuration_Trace source of channel 4", "type"=enum."U32", "rw"=enum."rw", "lowLimit"="0", "highLimit"="4294967295", "Default"="0x00", "Kommentart"=""}, {"ID"=594542603, "Name"="Trace configuration_Monitor source of channel 1", "type"=enum."U32", "rw"=enum."rw", "lowLimit"="0", "highLimit"="4294967295", "Default"="0x00", "Kommentart"=""}, {"ID"=594542604, "Name"="Trace configuration_Monitor source of channel 2", "type"=enum."U32", "rw"=enum."rw", "lowLimit"="0", "highLimit"="4294967295", "Default"="0x00", "Kommentart"=""}, {"ID"=594542605, "Name"="Trace configuration_Monitor source of channel 3", "type"=enum."U32", "rw"=enum."rw", "lowLimit"="0", "highLimit"="4294967295", "Default"="0x00", "Kommentart"=""}, {"ID"=594542606, "Name"="Trace configuration_Monitor source of channel 4", "type"=enum."U32", "rw"=enum."rw", "lowLimit"="0", "highLimit"="4294967295", "Default"="0x00", "Kommentart"=""}, {"ID"=594542607, "Name"="Trace configuration_Extended recorder mode", "type"=enum."U16", "rw"=enum."wo", "lowLimit"="0", "highLimit"="65535", "Default"="0x00", "Kommentart"=""}, {"ID"=594608128, "Name"="Trace buffer_Number 
